vi "Draw.vi"(8 "Error In":errorcluster, 10 "PictureIn":picture, 11 "object in":refnum<class "ObjectDecorator.lvclass">) -> (0 "Error Out":errorcluster, 2 "PictureOut":picture, 3 "object out":refnum<class "ObjectDecorator.lvclass">)   [LabVIEW 2020, in "ObjectDecorator.lvclass"]
uses:
  ObjectDecorator.lvclass
  ObjectDecorator.lvclass/ObjectDecorator.ctl
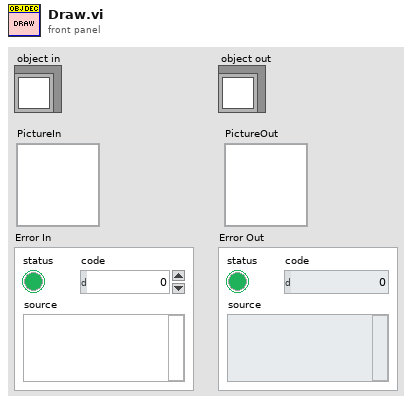
[diagram p1: front panel]
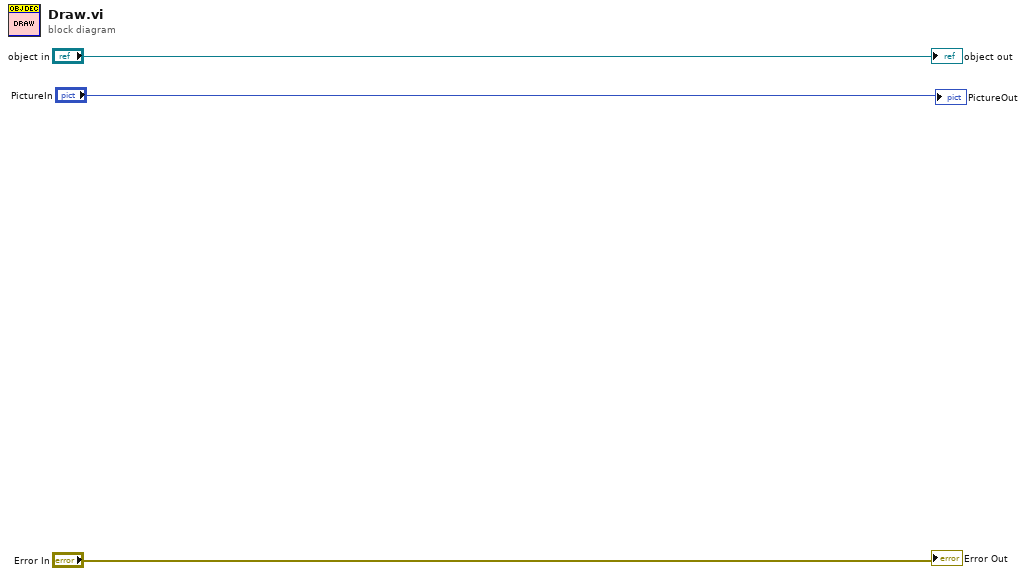
[diagram p0: block diagram]
diagram:
  "Error Out" <- "Error In"
  "object out" <- "object in"
  "PictureOut" <- "PictureIn"
